vi "Cleanup.vi"(8 "error in (no error)":errorcluster, 11 "TCP Stream in":refnum<class "TCP Stream.lvclass">) -> (0 "error out":errorcluster, 3 "TCP Stream out":refnum<class "TCP Stream.lvclass">)   [LabVIEW 2020, in "Stream-TCP.lvlib" / "TCP Stream.lvclass"]
uses:
  TCP Stream.lvclass
  TCP Stream.lvclass/TCP Stream.ctl
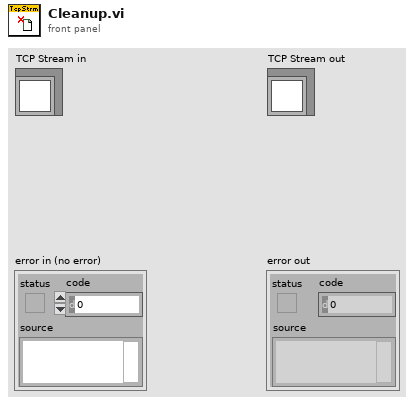
[diagram p1: front panel]
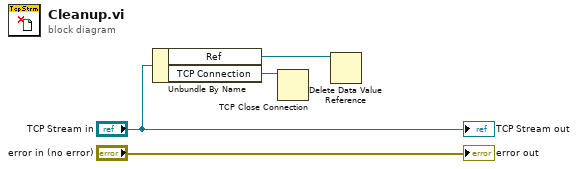
[diagram p0: block diagram]
diagram:
  n1 = Unbundle By Name("TCP Stream in") -> ("Ref"=w2:refnum<data-value>, "TCP Connection"=w3:refnum<k5>)
  n2 = TCP Close Connection(connection ID=w3) -> ()  [unwired: 2 in, 2 out]
  n3 = Delete Data Value Reference(data value reference=w2) -> ()  [unwired: 1 in, 2 out]
  "error out" <- "error in (no error)"
  "TCP Stream out" <- "TCP Stream in"
